vi "CWrapATC3DG_testAll.vi"() -> ()   [LabVIEW 2014]
uses:
  CWrapATC3DG.llb/systemCfg.ctl
  <vilib>/Analysis/Matrix/Datatypes/RealMatrix.ctl
  CWrapATC3DGlvlib/CWrapATC3DG.lvlib
  CWrapATC3DG.dll
  <vilib>/Analysis/Matrix/NI_Matrix.lvlib
panel:
  out "acWide":bool
  out "acNarrow":bool
  in  "setAC":bool
  out "alphaOnOff":i32
  out "dcValue":dbl
  out "i 2":i32
  out "i":i32
  in  "txANG":dbl[](array[numeric])=[0.1, 0.2, 0.3]
  out "oneSpeed[Hz]":dbl
  out "allSpeed[Hz]":dbl
  in  "stop":bool
  in  "sensorNum 5":i32
  out "quat":dbl[](array[numeric])
  out "pos":dbl[](array[numeric])
  in  "syncAll":bool
  out "allPQ 2":T1
  out "allPQ":T1
  out "pos":dbl[](array[numeric])
  out "ang":dbl[](array[numeric])
  out "posMat":T2
  out "posQuat":T2
  out "sensorCfg":T3
  out "DataFormatEnum 2":i32(ring) items=["no format selected", "short position", "short angles", "short matrix", "short quaternions", "short position angles", "shor position matrix", "short position quaternion", "double position", "double angles ", "double matrix", "double quaternions", "double position angles", "double position matrix", "double position quaternion", "double position time stamp", "double angles time stamp", "double matrix time stamp", "double quaternions time stamp", "double position angles time stamp", "double positio matrix time stamp", "double position quaternion time stamp", "double position time q", "double angles time q", "double matrix time q", "double quaternions time q", "double position angles time q", "double position matrix time q", "double position quaternions time q", "short all", "double all", "double all time stamp", "double all time stamp q", "double all time stamp q raw", "double position angles time q button", "double position matrix time q button", "double position quaternion time q button", "maximum format code"]
  in  "metricOn?":bool=TRUE
  out "offsetXYZ 2":dbl[](array[numeric])
  in  "sensorNum 4":i32=1
  out "offsetXYZ":dbl[](array[numeric])
  in  "sensorNum 3":i32
  out "xyzOn":i32
  out "angTx":dbl[](array[numeric])
  out "ang":dbl[](array[numeric])
  in  "ang":dbl[](array[numeric])=[0.1, 0.2, 0.3]
  in  "sensorNum":i32
  out "systemCfg":T4
  in  "resetOnInit":bool=TRUE
  out "ang":dbl[](array[numeric])
  in  "sensorNum 2":i32=1
  out "ang2":dbl[](array[numeric])
  in  "sensorNum":i32
  out "error out":errorcluster
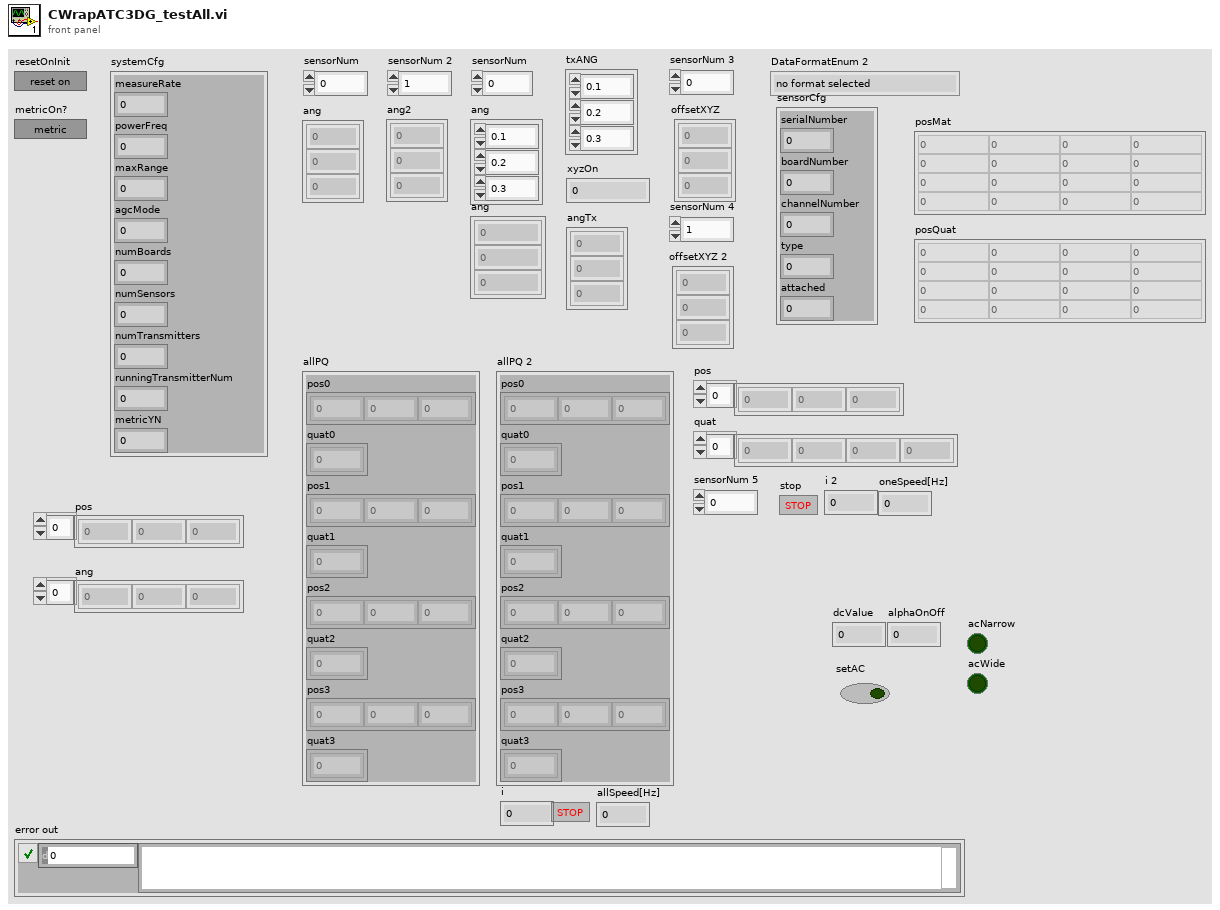
[diagram p1: front panel]
types:
  T1 = cluster{"pos0":dbl[], "quat0":dbl[], "pos1":dbl[], "quat1":dbl[], "pos2":dbl[], "quat2":dbl[], "pos3":dbl[], "quat3":dbl[]}
  T2 = typedef "NI_Matrix.lvlib/RealMatrix.ctl" = dbl[][]
  T3 = cluster{"serialNumber":u32, "boardNumber":u16, "channelNumber":u16, "type":u32, "attached":i32}
  T4 = typedef "systemCfg.ctl" = cluster{"measureRate":dbl, "powerFreq":dbl, "maxRange":dbl, "agcMode":i32, "numBoards":i32, "numSensors":i32, "numTransmitters":i32, "runningTransmitterNum":i32, "metricYN":i32}
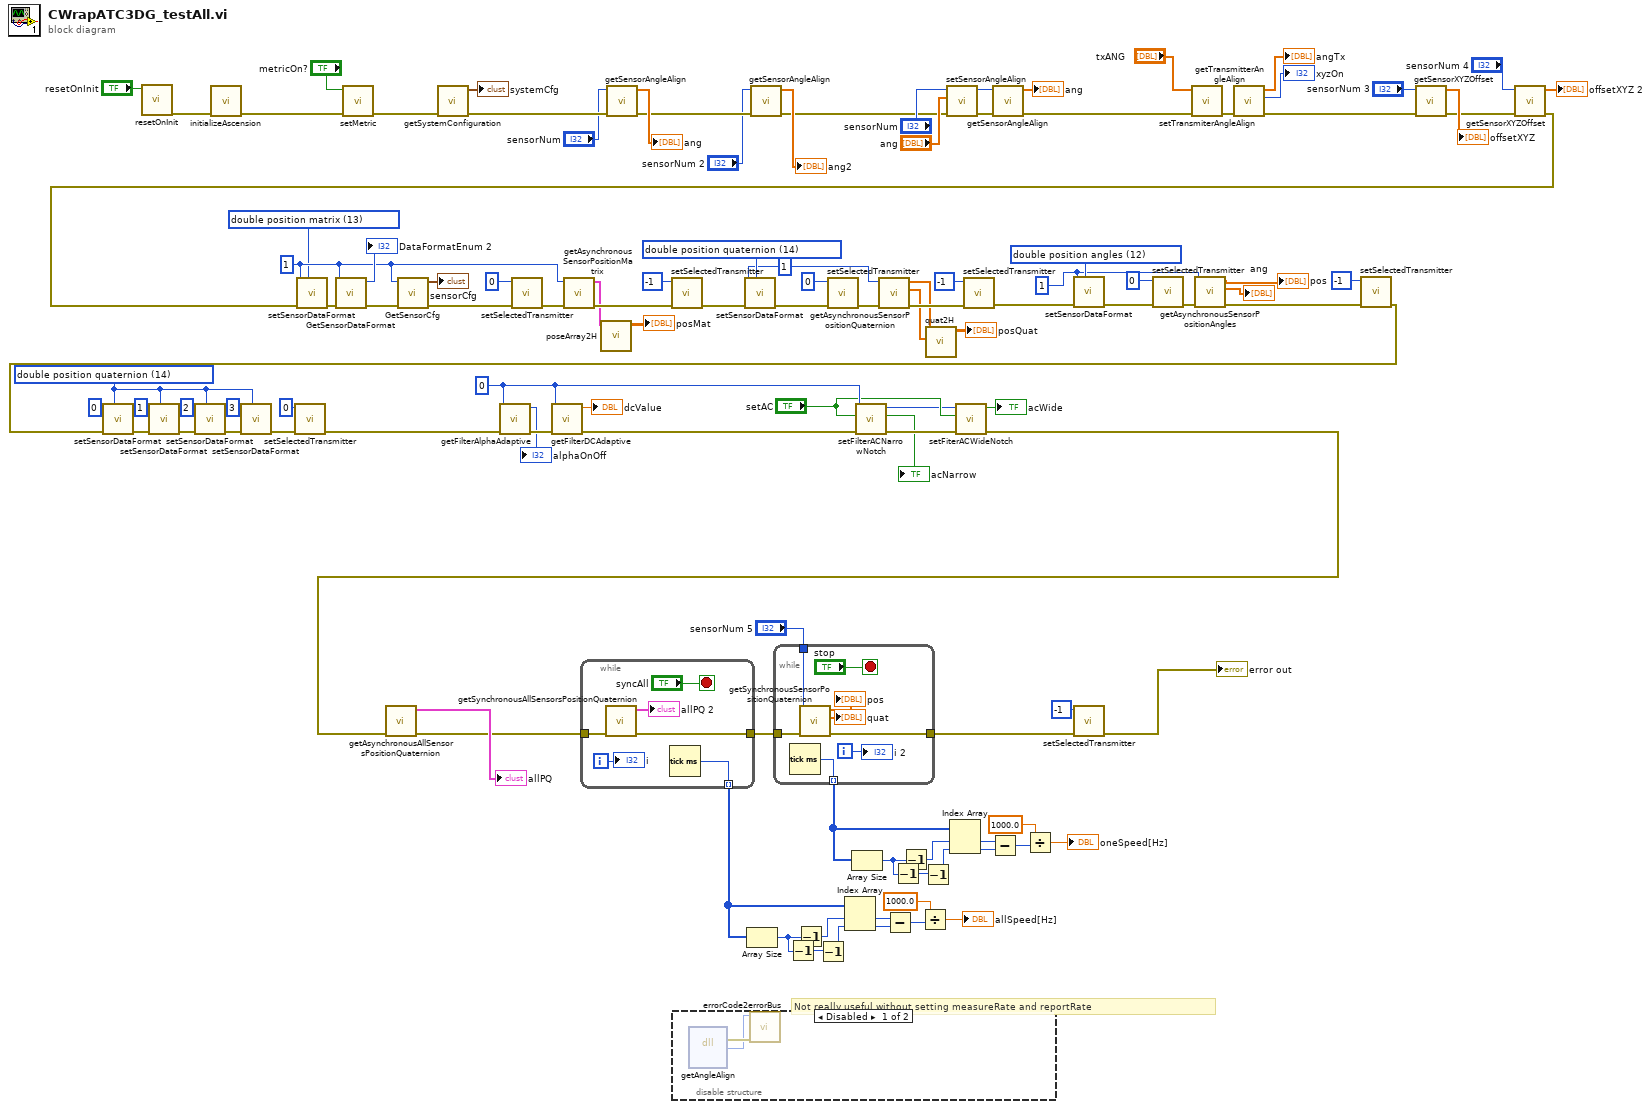
[diagram p0: block diagram]
diagram:
  w6 = 0 ("transmitterNum")
  w46 = 14 items=["no format selected"=0, "double position"=8, "double position angles"=12, "double position matrix"=13, "double position quaternion"=14] ("DataFormatType")
  w54 = 1 ("sensorNum")
  w62 = 12 items=["no format selected"=0, "double position"=8, "double position angles"=12, "double position matrix"=13, "double position quaternion"=14] ("DataFormatType")
  w75 = 14 items=["no format selected"=0, "double position"=8, "double position angles"=12, "double position matrix"=13, "double position quaternion"=14] ("DataFormatType")
  w64 = 1 ("sensorNum")
  w77 = 13 items=["no format selected"=0, "double position"=8, "double position angles"=12, "double position matrix"=13, "double position quaternion"=14] ("DataFormatType")
  w78 = 1 ("sensorNum")
  # "Not really useful without setting measureRate and reportRate"
  n1 = call "resetOnInit.vi"("reset01"="resetOnInit") -> ("error out"=w114:errorcluster)  [unwired: 10 in]
  n2 = call "initializeAscension.vi"("error in (no error)"=w114) -> ("error out"=w112:errorcluster)  [unwired: 10 in]
  n3 = call "setMetric.vi"("error in"=w112, "metricOn?"="metricOn?") -> ("error out"=w86:errorcluster)  [unwired: 9 in]
  n4 = call "getSystemConfiguration.vi"("error in (no error)"=w86) -> ("error out"=w101:errorcluster, "systemCfg"=→"systemCfg":T4)  [unwired: 9 in]
  n5 = call "getSensorAngleAlign.vi"("error in (no error)"=w101, "sensorNum"="sensorNum") -> ("error out"=w98:errorcluster, "ang"=→"ang":dbl[])  [unwired: 8 in]
  n6 = disable-structure shown="Disabled" {
    frame Disabled {
      n7 = dll-call lib="D:/20160401_inter2d_estimate/CWrapATC3DG/Release/CWrapATC3DG.*" fn="getAngleAlign"() -> (error out=w116:errorcluster, "errorCode"=w115:i32)  [unwired: 7 in, 1 out]
      n8 = call "errorCode2errorBus.vi"("error in (no error)"=w116, "errorCodeEnumIn"=w115) -> ()  [unwired: 9 in, 1 out]
    }
    frame Enabled {
    }
  }
  n9 = call "getSensorAngleAlign.vi"("error in (no error)"=w98, "sensorNum"="sensorNum 2") -> ("error out"=w95:errorcluster, "ang"=→"ang2":dbl[])  [unwired: 8 in]
  n10 = call "setSensorAngleAlign.vi"("error in"=w95, "angleAER"="ang", "sensorNum in"="sensorNum") -> ("error out"=w106:errorcluster, "sensorNum out"=w105:i32)  [unwired: 7 in]
  n11 = call "getSensorAngleAlign.vi"("error in (no error)"=w106, "sensorNum"=w105) -> ("error out"=w15:errorcluster, "ang"=→"ang":dbl[])  [unwired: 8 in]
  n12 = call "setTransmiterAngleAlign.vi"("error in"=w15, "alignTx[rad]"="txANG") -> ("error out"=w14:errorcluster)  [unwired: 9 in]
  n13 = call "getTransmitterAngleAlign.vi"("error in"=w14) -> ("error out"=w92:errorcluster, "xyzOn"=→"xyzOn":i32, "angTx"=→"angTx":dbl[])  [unwired: 8 in]
  n14 = call "getSensorXYZOffset.vi"("error in"=w92, "sensorNum"="sensorNum 3") -> ("error out"=w88:errorcluster, "offsetXYZ"=→"offsetXYZ":dbl[])  [unwired: 8 in]
  n15 = call "getSensorXYZOffset.vi"("error in"=w88, "sensorNum"="sensorNum 4") -> ("error out"=w111:errorcluster, "offsetXYZ"=→"offsetXYZ 2":dbl[])  [unwired: 8 in]
  n16 = call "setSensorDataFormat.vi"("DataFormatType"=w77, "error in"=w111, "sensorNum"=w78) -> ("error out"=w84:errorcluster)  [unwired: 8 in]
  n17 = call "GetSensorDataFormat.vi"("error in (no error)"=w84, "channelNum"=w78) -> ("error out"=w110:errorcluster, "DataFormatEnum 2"=→"DataFormatEnum 2":i32)  [unwired: 8 in]
  n18 = call "GetSensorCfg.vi"("error in (no error)"=w110, "channelNum"=w78) -> ("error out"=w83:errorcluster, "sensorCfg"=→"sensorCfg":T3)  [unwired: 7 in]
  n19 = call "setSelectedTransmitter.vi"("error in (no error)"=w83, "transmitterNum"=0) -> ("error out"=w81:errorcluster)  [unwired: 9 in]
  n20 = call "getAsynchronousSensorPositionMatrix.vi"("error in (no error)"=w81, "sensorNum"=w78) -> ("error out"=w80:errorcluster, "pose"=w66:cluster{"position":dbl[], "matrix":dbl[]})  [unwired: 8 in]
  n21 = call "poseArray2H.vi"("poseArray"=w66) -> ("poseH"=→"posMat":dbl[][])  [unwired: 10 in]
  n22 = call "setSelectedTransmitter.vi"("error in (no error)"=w80, "transmitterNum"=-1) -> ("error out"=w76:errorcluster)  [unwired: 9 in]
  n23 = call "setSensorDataFormat.vi"("DataFormatType"=w75, "error in"=w76, "sensorNum"=w64) -> ("error out"=w72:errorcluster)  [unwired: 8 in]
  n24 = call "setSelectedTransmitter.vi"("error in (no error)"=w72, "transmitterNum"=0) -> ("error out"=w71:errorcluster)  [unwired: 9 in]
  n25 = call "getAsynchronousSensorPositionQuaternion.vi"("error in"=w71, "sensorNum"=w64) -> ("error out"=w70:errorcluster, "quat"=w68:dbl[], "pos"=w69:dbl[])  [unwired: 7 in]
  n26 = call "quat2H.vi"("quat"=w68, "pos"=w69) -> ("H"=→"posQuat":T2)  [unwired: 9 in]
  n27 = call "setSelectedTransmitter.vi"("error in (no error)"=w70, "transmitterNum"=-1) -> ("error out"=w63:errorcluster)  [unwired: 9 in]
  n28 = call "setSensorDataFormat.vi"("DataFormatType"=w62, "error in"=w63, "sensorNum"=w54) -> ("error out"=w59:errorcluster)  [unwired: 8 in]
  n29 = call "setSelectedTransmitter.vi"("error in (no error)"=w59, "transmitterNum"=0) -> ("error out"=w56:errorcluster)  [unwired: 9 in]
  n30 = call "getAsynchronousSensorPositionAngles.vi"("error in"=w56, "sensorNum"=w54) -> ("error out"=w55:errorcluster, "ang"=→"ang":dbl[], "pos"=→"pos":dbl[])  [unwired: 7 in]
  n31 = call "setSelectedTransmitter.vi"("error in (no error)"=w55, "transmitterNum"=-1) -> ("error out"=w45:errorcluster)  [unwired: 9 in]
  n32 = call "setSensorDataFormat.vi"("DataFormatType"=w46, "error in"=w45, "sensorNum"=0) -> ("error out"=w49:errorcluster)  [unwired: 8 in]
  n33 = call "setSensorDataFormat.vi"("DataFormatType"=w46, "error in"=w49, "sensorNum"=1) -> ("error out"=w48:errorcluster)  [unwired: 8 in]
  n34 = call "setSensorDataFormat.vi"("DataFormatType"=w46, "error in"=w48, "sensorNum"=2) -> ("error out"=w47:errorcluster)  [unwired: 8 in]
  n35 = call "setSensorDataFormat.vi"("DataFormatType"=w46, "error in"=w47, "sensorNum"=3) -> ("error out"=w44:errorcluster)  [unwired: 8 in]
  n36 = call "setSelectedTransmitter.vi"("error in (no error)"=w44, "transmitterNum"=0) -> ("error out"=w3:errorcluster)  [unwired: 9 in]
  n37 = call "getFilterAlphaAdaptive.vi"("error in"=w3, "sensorNum"=w6) -> ("error out"=w12:errorcluster, "acOnOff"=→"alphaOnOff":i32)  [unwired: 5 in, 3 out]
  n38 = call "getFilterDCAdaptive.vi"("error in"=w12, "sensorNum"=w6) -> ("error out"=w9:errorcluster, "dcValue"=→"dcValue":dbl)  [unwired: 8 in]
  n39 = call "setFilterACNarrowNotch.vi"("error in"=w9, "setAC"="setAC", "sensorNum"=w6) -> ("error out"=w8:errorcluster, "acOnOff"=→"acNarrow":bool, "sensorNum"=w1:i32)  [unwired: 6 in]
  n40 = call "setFiterACWideNotch.vi"("error in"=w8, "acOnOff"="setAC", "sensorNum"=w1) -> ("error out"=w7:errorcluster, "acOnOff"=→"acWide":bool)  [unwired: 7 in]
  n41 = call "getAsynchronousAllSensorsPositionQuaternion.vi"("error in"=w7) -> ("error out"=w41:errorcluster, "allPQ"=→"allPQ":T1)  [unwired: 9 in]
  n42 = while {
    tunnel: w41 -> [w121]
    tunnel: [w119] -> w37
    tunnel: [w118] -> w32 mode=indexing
    i -> [w117]
    stop <- "syncAll" stop-if-true
    n43 = call "getSynchronousAllSensorsPositionQuaternion.vi"("error in"=w121) -> ("error out"=w119:errorcluster, "syncPQ"=→"allPQ 2":T1)  [unwired: 9 in]
    n44 = Tick Count (ms)() -> (millisecond timer value=w118:u32)
    "i" <- w117
  }
  n45 = Array Size(array=w32) -> (size(s)=w36:i32)
  n46 = while {
    tunnel: w37 -> [w129]
    tunnel: [w130] -> w38
    tunnel: [w125] -> w17 mode=indexing
    tunnel: "sensorNum 5" -> [w124]
    i -> [w123]
    stop <- "stop" stop-if-true
    n47 = Tick Count (ms)() -> (millisecond timer value=w125:u32)
    n48 = call "getSynchronousSensorPositionQuaternion.vi"("error in"=w129, "sensorNum"=w124) -> ("error out"=w130:errorcluster, "quat"=→"quat":dbl[], "pos"=→"pos":dbl[])  [unwired: 7 in]
    "i 2" <- w123
  }
  n49 = Decrement(x=w36) -> (x-1=w35:i32)
  n50 = Decrement(x=w36) -> (x-1=w34:i32)
  n51 = Decrement(x=w35) -> (x-1=w33:i32)
  n52 = Index Array(array=w32, index #1=w34, index #2=w33) -> (element #1=w30:u32, element #2=w31:u32)
  n53 = Array Size(array=w17) -> (size(s)=w26:i32)
  n54 = Subtract(x=w30, y=w31) -> (x-y=w29:u32)
  n55 = Decrement(x=w26) -> (x-1=w25:i32)
  n56 = Decrement(x=w26) -> (x-1=w24:i32)
  n57 = Divide(x=1000.0, y=w29) -> (x/y=→"allSpeed[Hz]":dbl)
  n58 = Decrement(x=w25) -> (x-1=w23:i32)
  n59 = Index Array(array=w17, index #1=w24, index #2=w23) -> (element #1=w21:u32, element #2=w22:u32)
  n60 = Subtract(x=w21, y=w22) -> (x-y=w20:u32)
  n61 = Divide(x=1000.0, y=w20) -> (x/y=→"oneSpeed[Hz]":dbl)
  n62 = call "setSelectedTransmitter.vi"("error in (no error)"=w38, "transmitterNum"=-1) -> ("error out"=→"error out":errorcluster)  [unwired: 9 in]
